vi "Read Single Device.vi"(6 "Index":i32, 7 "Section":string, 8 "error in (no error)":errorcluster, 9 "Key Names":string[](array[string]), 11 "refnum":T1) -> (0 "error out":errorcluster, 1 "Remaining Key Names":string[](array[string]), 3 "refnum out":T1, 5 "Device":refnum<class "Device.lvclass">)   [LabVIEW 2020, in "PicoG-App.lvlib" / "App.lvclass"]
uses:
  App.lvclass
  <vilib>/Utility/config.llb/NI_LVConfig.lvlib
  <vilib>/Utility/config.llb/Read Key (String).vi
  Device/Device.lvclass
  Device/Device Key.ctl
  Builds/picoG/ppl/PicoG-Core.lvlibp/PicoG-Processor/PicoG-Core/DeployResource/DeployResource.lvclass
  Builds/picoG/ppl/PicoG-Core.lvlibp/PicoG-Processor/PicoG-Core/DeployResource/Config Item.ctl
  <vilib>/Utility/config.llb/Config Data RefNum.ctl
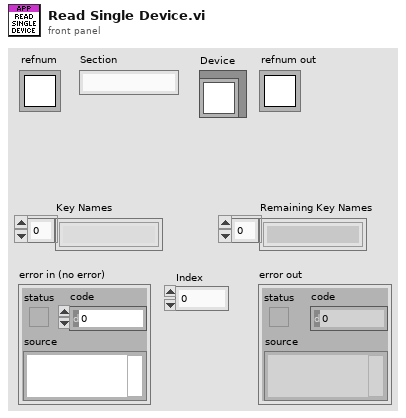
[diagram p1: front panel]
types:
  T1 = typedef "NI_LVConfig.lvlib/Config Data RefNum.ctl" = refnum<k1>
  T2 = typedef "PicoG-App.lvlib/Device.lvclass/Device Key.ctl" = cluster{"Platform":string, "Board":string, "ID":string}
  T3 = typedef "PicoG-Core.lvlibp/DeployResource.lvclass/Config Item.ctl" = cluster{"Key":string, "Value":string}
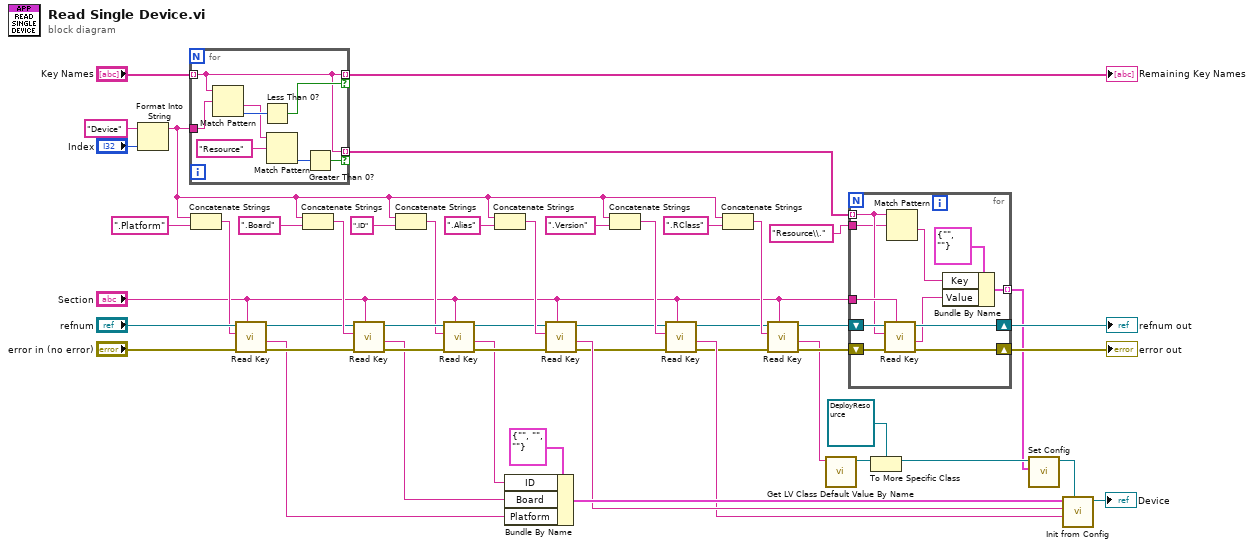
[diagram p0: block diagram]
diagram:
  n1 = Format Into String(initial string="Device", "Index") -> (resulting string=w16:string)  [unwired: 2 in, 1 out]
  n2 = for {
    tunnel: "Key Names" -> [w52] mode=indexing
    tunnel: w16 -> [w58]
    tunnel: [w52] -> w48 mode=indexing if=w56
    tunnel: [w52] -> w19 mode=indexing if=w51
    n3 = Match Pattern(string=w52, regular expression=w58) -> (after substring=w55:string, offset past match=w57:i32)  [unwired: 1 in, 2 out]
    n4 = Less Than 0?(x=w57) -> (x < 0?=w56:bool)
    n5 = Match Pattern(string=w55, regular expression="Resource") -> (offset past match=w53:i32)  [unwired: 1 in, 3 out]
    n6 = Greater Than 0?(x=w53) -> (x > 0?=w51:bool)
  }
  "Remaining Key Names" <- w48
  n7 = Concatenate Strings(w16, ".Platform" ("string")) -> (w40:string)
  n8 = call-poly <vilib>:"Read Key.vi"("section"="Section", "error in (no error)"="error in (no error)", "key"=w40, "refnum"="refnum") -> ("error out"=w37:errorcluster, "value"=w28:string, "refnum out"=w38:T1)  [unwired: 4 in, 1 out]
  n9 = Concatenate Strings(w16, ".Board" ("string")) -> (w39:string)
  n10 = call-poly <vilib>:"Read Key.vi"("section"="Section", "error in (no error)"=w37, "key"=w39, "refnum"=w38) -> ("error out"=w35:errorcluster, "value"=w27:string, "refnum out"=w36:T1)  [unwired: 4 in, 1 out]
  n11 = Concatenate Strings(w16, ".ID" ("string")) -> (w34:string)
  n12 = call-poly <vilib>:"Read Key.vi"("section"="Section", "error in (no error)"=w35, "key"=w34, "refnum"=w36) -> ("error out"=w31:errorcluster, "value"=w26:string, "refnum out"=w32:T1)  [unwired: 4 in, 1 out]
  n13 = Concatenate Strings(w16, ".Alias" ("string")) -> (w33:string)
  n14 = Bundle By Name(cluster=T2 {"Platform"="", "Board"="", "ID"=""} ("Device Key"), "ID"=w26, "Board"=w27, "Platform"=w28) -> (w29:T2)
  n15 = call-poly <vilib>:"Read Key.vi"("section"="Section", "error in (no error)"=w31, "key"=w33, "refnum"=w32) -> ("error out"=w20:errorcluster, "value"=w25:string, "refnum out"=w21:T1)  [unwired: 4 in, 1 out]
  n16 = Concatenate Strings(w16, ".Version" ("string")) -> (w22:string)
  n17 = call-poly <vilib>:"Read Key.vi"("section"="Section", "error in (no error)"=w20, "key"=w22, "refnum"=w21) -> ("error out"=w13:errorcluster, "value"=w24:string, "refnum out"=w14:T1)  [unwired: 4 in, 1 out]
  n18 = Concatenate Strings(w16, ".RClass" ("string")) -> (w15:string)
  n19 = call-poly <vilib>:"Read Key.vi"("section"="Section", "error in (no error)"=w13, "key"=w15, "refnum"=w14) -> ("error out"=w11:errorcluster, "value"=w9:string, "refnum out"=w10:T1)  [unwired: 4 in, 1 out]
  n20 = call <vilib>:"Get LV Class Default Value By Name.vi"("class name"=w9) -> ("object"=w8:refnum<class>)  [unwired: 9 in, 1 out]
  n21 = for {
    shift-right: [w65] -> w4
    shift-left: w11 -> [w69]
    shift-right: [w66] -> w5
    shift-left: w10 -> [w68]
    tunnel: "Section" -> [w67]
    tunnel: w19 -> [w64] mode=indexing
    tunnel: "Resource\\." ("regular expression") -> [w63]
    tunnel: [w59] -> w3 mode=indexing
    n22 = call-poly <vilib>:"Read Key.vi"("section"=w67, "error in (no error)"=w69, "key"=w64, "refnum"=w68) -> ("error out"=w65:errorcluster, "value"=w61:string, "refnum out"=w66:T1)  [unwired: 4 in, 1 out]
    n23 = Match Pattern(string=w64, regular expression=w63) -> (after substring=w60:string)  [unwired: 1 in, 3 out]
    n24 = Bundle By Name(cluster=T3 {"Key"="", "Value"=""} ("Config Item"), "Key"=w60, "Value"=w61) -> (w59:T3)
  }
  "error out" <- w4
  "refnum out" <- w5
  n25 = To More Specific Class(target class=refnum<class "DeployResource.lvclass"> refnum ("Resource"), reference=w8) -> (specific class reference=w6:refnum<class "DeployResource.lvclass">)  [unwired: 1 in, 1 out]
  n26 = call "Set Config.vi"("Config"=w3, "DeployResource in"=w6) -> ("DeployResource out"=w2:refnum<class "DeployResource.lvclass">)  [unwired: 8 in, 1 out]
  n27 = call "Init from Config.vi"("Resource"=w2, "Version"=w24, "Alias"=w25, "Device Key"=w29) -> ("Device out"=→"Device":refnum<class "Device.lvclass">)  [unwired: 6 in, 1 out]
